vi "InitialDelayCountdown_DP_Ver1.0.vi"(1 "Temp. Display Ref Array":refnum<vi>[](array[refnum]), 9 "output cluster":T1={"Main Sweep"=0, "Steps Config:"={"total points:"=0, "Step Delay (s)"=0.0, "Ini Delay (s)"=0.0, "# of steps:"=0}, "Temperature Control (ITC 503):"={"GPIB ADR"=0, "Change Heater?"={"Heater?"=FALSE, "Heater"=0}, "Change Temp?"={"Change T?"=FALSE, "Set T (K)"=0.0}, "Cluster"={"Heat Auto?"=FALSE, "Manual Heat?"=FALSE, "Heater (%)"=0.0}, "Change PID?"={"Change PID?"=FALSE, "P"=0.0, "I"=0.0, "D"=0.0}, "Change Para?"=FALSE, "Sensor"=1}, "Temperature Control (LS 340):"={"GPIB ADR"=0, "From (K)"=0.0, "To (K)"=0.0, "Rate (K/min)"=0.0, "Delta T (0.08K)"=0.0, "Temp. Header"="", "T Display Control"={"Ch B"=FALSE, "Ch C"=FALSE, "Ch D"=FALSE}}, "Magnet Control (IPS 120-10)"={"Action"=0, "Standby (s)"=0.0, "Heater on (s)"=0.0, "Sweep Setup "=[], "GPIB ADR"=0, "Change Para?"=FALSE}, "Keithley 6221 :"=[], "Measuring Instruments : "=[], "Lock-In SR7265 :"=[], "Deascription of \nthis measurement"="", "Instruments Config:"=[], "LS372 Bridge : 2"=[{"GPIB"=0, "Excitation"=0, "Autorange?"=FALSE, "Range"=0, "Current"=0, "Voltage"=0, "DataHeader"="Rx;Ry"}], "Magnet Control (CS4) 2"={"Action"=1, "Standby (s)"=0.0, "Heater on (s)"=300.0, "Sweep Setup "=[], "GPIB ADR"=0, "Change Para?"=FALSE}} {"Magnet Control (CS4) 2"."GPIB ADR" items=["None"=0, "25"=25]; "Magnet Control (CS4) 2"."Sweep Setup"."Rate in Range (T/min)" min=0.001 max=0.5 step=0.001; "Magnet Control (CS4) 2"."Sweep Setup"."Hold(min)" min=0.0; "Magnet Control (CS4) 2"."Sweep Setup"."Set Point (T)" min=-9.0 max=9.0 step=0.001; "Magnet Control (CS4) 2"."Action" items=["Up", "Down", "Pause", "Zero"]; "LS372 Bridge : 2"."Voltage" items=["2.00 uV"=1, "6.32 uV"=2, "20.0 uV"=3, "63.2 uV"=4, "200 uV"=5, "632 uV"=6, "2.0 mV"=7, "6.32 mV"=8]; "LS372 Bridge : 2"."Current" items=["1.00 pA"=1, "3.16 pA"=2, "10.0 pA"=3, "31.6 pA"=4, "100 pA"=5, "316 pA"=6, "1.00 nA"=7, "3.16 nA"=8, "10 nA"=9, "31.6 nA"=10, "100 nA"=11, "316 nA"=12, "1.00 uA"=13, "3.16 uA"=14, "10.0 uA"=15, "31.6 uA"=16, "100 uA"=17, "316 uA"=18, "1.00 mA"=19, "3.16 mA"=20, "10.0 mA"=21, "31.6 mA"=22]; "LS372 Bridge : 2"."Range" items=["2.0 m"=1, "6.32 m"=2, "20.0 m"=3, "63.2 m"=4, "200 m"=5, "632 m"=6, "2.00"=7, "6.32"=8, "20.0"=9, "63.2"=10, "200"=11, "632"=12, "2.00 k"=13, "6.32 k"=14, "20.0 k"=15, "63.2 k"=16, "200 k"=17, "632 k"=18, "2.00 M"=19, "6.32 M"=20, "20.0 M"=21, "63.2 M"=22]; "LS372 Bridge : 2"."Excitation" items=["Voltage", "Current"]; "LS372 Bridge : 2"."GPIB" items=["None"=0, "9"=9]; "Main Sweep" items=["Time", "DC Current", "Delta Current", "Pulse Delta Current", "Sine Current", "Lock-in Vosc"]; "Temperature Control (ITC 503):"."Sensor" items=["T2", "T3"]; "Magnet Control (IPS 120-10)"."Action" items=["Hold", "To Set point", "To Zero", "Clamp"]; "Keithley 6221 :"."Sweep Mode" items=["Linear", "Log", "Exp", "Inverse", "Manual"]}, 11 "error in":errorcluster, 12 "B Field Display Tex Array":refnum<vi>[](array[refnum])) -> (4 "Stay duration pts":dbl[](array[numeric]), 8 "2D Array of DC Source or Lock-In Ctrl Run Cluster":cluster{"GPIB ADR":u16, "DC St. Pt.":dbl}[][](array[cluster]), 10 "output cluster 2":T1={"Main Sweep"=0, "Steps Config:"={"total points:"=0, "Step Delay (s)"=0.0, "Ini Delay (s)"=0.0, "# of steps:"=0}, "Temperature Control (ITC 503):"={"GPIB ADR"=0, "Change Heater?"={"Heater?"=FALSE, "Heater"=0}, "Change Temp?"={"Change T?"=FALSE, "Set T (K)"=0.0}, "Cluster"={"Heat Auto?"=FALSE, "Manual Heat?"=FALSE, "Heater (%)"=0.0}, "Change PID?"={"Change PID?"=FALSE, "P"=0.0, "I"=0.0, "D"=0.0}, "Change Para?"=FALSE, "Sensor"=1}, "Temperature Control (LS 340):"={"GPIB ADR"=0, "From (K)"=0.0, "To (K)"=0.0, "Rate (K/min)"=0.0, "Delta T (0.08K)"=0.0, "Temp. Header"="", "T Display Control"={"Ch B"=FALSE, "Ch C"=FALSE, "Ch D"=FALSE}}, "Magnet Control (IPS 120-10)"={"Action"=0, "Standby (s)"=0.0, "Heater on (s)"=0.0, "Sweep Setup "=[], "GPIB ADR"=0, "Change Para?"=FALSE}, "Keithley 6221 :"=[], "Measuring Instruments : "=[], "Lock-In SR7265 :"=[], "Deascription of \nthis measurement"="", "Instruments Config:"=[], "LS372 Bridge : 2"=[{"GPIB"=0, "Excitation"=0, "Autorange?"=FALSE, "Range"=0, "Current"=0, "Voltage"=0, "DataHeader"="Rx;Ry"}], "Magnet Control (CS4) 2"={"Action"=1, "Standby (s)"=0.0, "Heater on (s)"=300.0, "Sweep Setup "=[], "GPIB ADR"=0, "Change Para?"=FALSE}} {"Magnet Control (CS4) 2"."GPIB ADR" items=["None"=0, "25"=25]; "Magnet Control (CS4) 2"."Sweep Setup"."Rate in Range (T/min)" min=0.001 max=0.5 step=0.001; "Magnet Control (CS4) 2"."Sweep Setup"."Hold(min)" min=0.0; "Magnet Control (CS4) 2"."Sweep Setup"."Set Point (T)" min=-9.0 max=9.0 step=0.001; "Magnet Control (CS4) 2"."Action" items=["Up", "Down", "Pause", "Zero"]; "LS372 Bridge : 2"."Voltage" items=["2.00 uV"=1, "6.32 uV"=2, "20.0 uV"=3, "63.2 uV"=4, "200 uV"=5, "632 uV"=6, "2.0 mV"=7, "6.32 mV"=8]; "LS372 Bridge : 2"."Current" items=["1.00 pA"=1, "3.16 pA"=2, "10.0 pA"=3, "31.6 pA"=4, "100 pA"=5, "316 pA"=6, "1.00 nA"=7, "3.16 nA"=8, "10 nA"=9, "31.6 nA"=10, "100 nA"=11, "316 nA"=12, "1.00 uA"=13, "3.16 uA"=14, "10.0 uA"=15, "31.6 uA"=16, "100 uA"=17, "316 uA"=18, "1.00 mA"=19, "3.16 mA"=20, "10.0 mA"=21, "31.6 mA"=22]; "LS372 Bridge : 2"."Range" items=["2.0 m"=1, "6.32 m"=2, "20.0 m"=3, "63.2 m"=4, "200 m"=5, "632 m"=6, "2.00"=7, "6.32"=8, "20.0"=9, "63.2"=10, "200"=11, "632"=12, "2.00 k"=13, "6.32 k"=14, "20.0 k"=15, "63.2 k"=16, "200 k"=17, "632 k"=18, "2.00 M"=19, "6.32 M"=20, "20.0 M"=21, "63.2 M"=22]; "LS372 Bridge : 2"."Excitation" items=["Voltage", "Current"]; "LS372 Bridge : 2"."GPIB" items=["None"=0, "9"=9]; "Main Sweep" items=["Time", "DC Current", "Delta Current", "Pulse Delta Current", "Sine Current", "Lock-in Vosc"]; "Temperature Control (ITC 503):"."Sensor" items=["T2", "T3"]; "Magnet Control (IPS 120-10)"."Action" items=["Hold", "To Set point", "To Zero", "Clamp"]; "Keithley 6221 :"."Sweep Mode" items=["Linear", "Log", "Exp", "Inverse", "Manual"]}, 15 "error out":errorcluster)   [LabVIEW 2012]
doc: "Initial Delay for LS336 Temperature controller"
panel:
  in  "Initial Delay (sec)":dbl=25.0
  in  "Skip":bool
  out "Time Count down":dbl format="%02d"
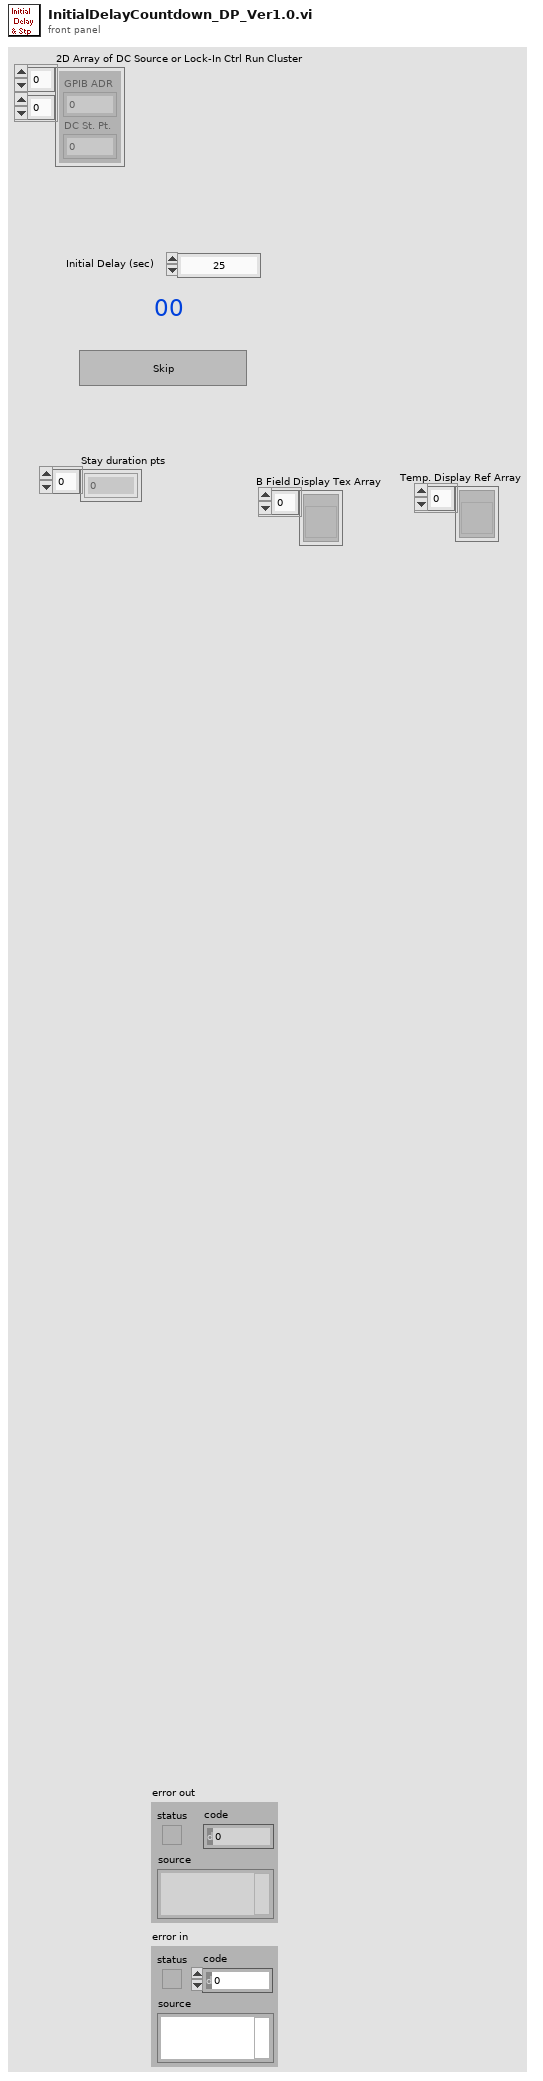
[diagram p1: front panel]
types:
  T1 = cluster{"Main Sweep":u8, "Steps Config:":cluster{"total points:":u32, "Step Delay (s)":dbl, "Ini Delay (s)":dbl, "# of steps:":u32}, "Temperature Control (ITC 503):":cluster{"GPIB ADR":u16, "Change Heater?":cluster{"Heater?":bool, "Heater":u8}, "Change Temp?":cluster{"Change T?":bool, "Set T (K)":dbl}, "Cluster":cluster{"Heat Auto?":bool, "Manual Heat?":bool, "Heater (%)":dbl}, "Change PID?":cluster{"Change PID?":bool, "P":dbl, "I":dbl, "D":dbl}, "Change Para?":bool, "Sensor":u16}, "Temperature Control (LS 340):":cluster{"GPIB ADR":u16, "From (K)":dbl, "To (K)":dbl, "Rate (K/min)":dbl, "Delta T (0.08K)":dbl, "Temp. Header":string, "T Display Control":cluster{"Ch B":bool, "Ch C":bool, "Ch D":bool}}, "Magnet Control (IPS 120-10)":cluster{"Action":u16, "Standby (s)":dbl, "Heater on (s)":dbl, "Sweep Setup ":cluster{"Set Point (T)":dbl, "Set Rate(T/min)":dbl, "Hold(min)":dbl}[], "GPIB ADR":u16, "Change Para?":bool}, "Keithley 6221 :":cluster{"Delta mode":bool, "Const I":bool, "Pulse Delta mode":bool, "Sine Wave Mode":bool, "From I_HI (A)":dbl, "From I (A)":dbl, "I_LO (A)":dbl, "From I_H (A)":dbl, "I_L (A)":dbl, "Freq (Hz)":dbl, "From I_Sin (A)":dbl, "DC Offset (A)":dbl, "Delay Time (s)":dbl, "Pulse Width (s)":dbl, "Delay (s)":dbl, "To I (A)":dbl, "ASymmetric?":bool, "To I_HI (A)":dbl, "To I_H (A)":dbl, "To I_Sin (A)":dbl, "GPIB ADR":u16, "Sweep Mode":u8, "Delta Unit":string, "2182A range (V)":dbl, "6221 Compliance (V)":dbl}[], "Measuring Instruments : ":cluster{"GPIB Bus":dbl, "GPIB Addr":dbl, "Instrument":enum16{"None", "HP34401DMM", "Lockin 7265", "HP3456/7A", "HP3478A", "HP3325FG", "Keithley2182A"}, "Instru Header":string}[], "Lock-In SR7265 :":cluster{"GPIB ADR":u16, "From":dbl, "To":dbl, "Header(;)":string, "Sweep Mode":u8}[], "Deascription of \nthis measurement":string, "Instruments Config:":string[][], "LS372 Bridge : 2":cluster{"GPIB":u16, "Excitation":u16, "Autorange?":bool, "Range":u16, "Current":u16, "Voltage":u16, "DataHeader":string}[], "Magnet Control (CS4) 2":cluster{"Action":u16, "Standby (s)":dbl, "Heater on (s)":dbl, "Sweep Setup ":cluster{"Set Point (T)":dbl, "Hold(min)":dbl, "Rate in Range (T/min)":dbl[]}[], "GPIB ADR":u16, "Change Para?":bool}}
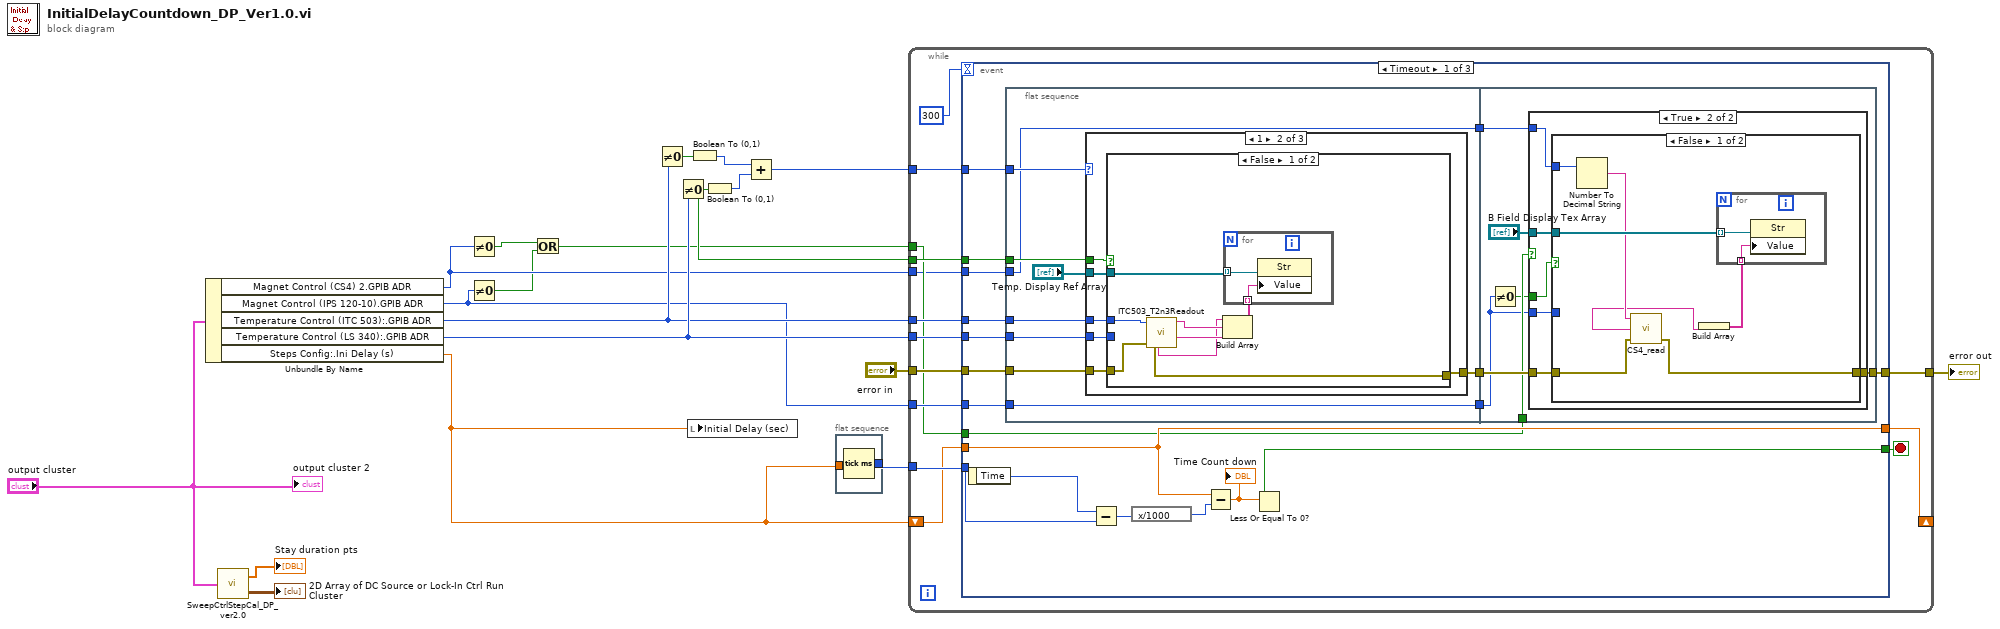
[diagram p0: block diagram]
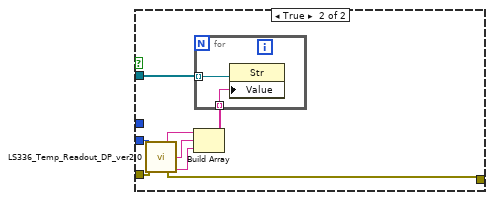
[diagram p3: hidden frame]
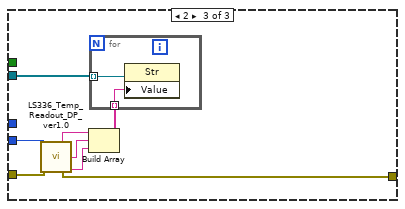
[diagram p4: hidden frame]
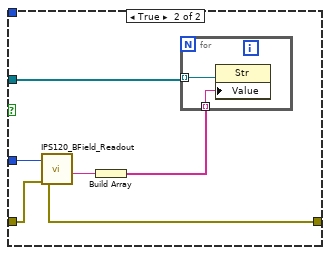
[diagram p6: hidden frame]
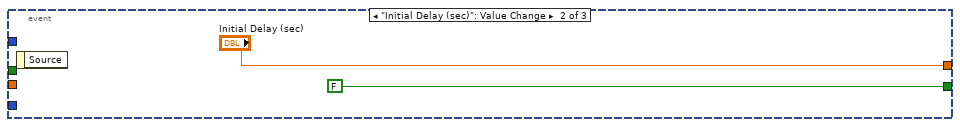
[diagram p7: hidden frame]
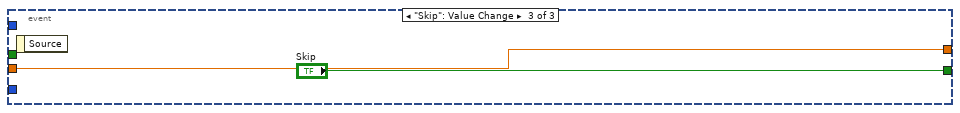
[diagram p8: hidden frame]
diagram:
  n1 = Unbundle By Name("output cluster") -> ("Magnet Control (CS4) 2.GPIB ADR"=w4:u16, "Magnet Control (IPS 120-10).GPIB ADR"=w5:u16, "Temperature Control (ITC 503):.GPIB ADR"=w8:u16, "Temperature Control (LS 340):.GPIB ADR"=w14:u16, "Steps Config:.Ini Delay (s)"=w15:dbl)
  n2 = call "SweepCtrlStepCal_DP_ver2.0.vi"("output cluster"="output cluster") -> ("Stay duration pts"=→"Stay duration pts":dbl[], "2D Array of DC Source or Lock-In Ctrl Run Cluster"=→"2D Array of DC Source or Lock-In Ctrl Run Cluster":cluster{"GPIB ADR":u16, "DC St. Pt.":dbl}[][])
  n3 = Not Equal To 0?(x=w4) -> (x != 0?=w3:bool)
  n4 = Not Equal To 0?(x=w5) -> (x != 0?=w2:bool)
  n5 = Or(x=w3, y=w2) -> (x .or. y?=w1:bool)
  n6 = Not Equal To 0?(x=w8) -> (x != 0?=w13:bool)
  n7 = Not Equal To 0?(x=w14) -> (x != 0?=w9:bool)
  n8 = local write "Initial Delay (sec)"(w15) -> ()
  n9 = Boolean To (0,1)(Boolean=w13) -> (0, 1=w11:i16)
  n10 = Boolean To (0,1)(Boolean=w9) -> (0, 1=w12:i16)
  n11 = Add(x=w11, y=w12) -> (x+y=w10:i16)
  n12 = flat-sequence {
    tunnel: [w20] -> w18
    tunnel: w15 -> [_]
    frame #0 {
      n13 = Tick Count (ms)() -> (millisecond timer value=w20:u32)
    }
  }
  n14 = while {
    tunnel: w18 -> [w34]
    shift-right: [w31] -> _
    shift-left: w15 -> [w32]
    tunnel: "error in" -> [w30]
    tunnel: [w29] -> w16
    tunnel: w14 -> [w28]
    tunnel: w10 -> [w26]
    tunnel: w9 -> [w25]
    tunnel: w8 -> [w24]
    tunnel: w5 -> [w23]
    tunnel: w4 -> [w21]
    tunnel: w1 -> [w22]
    stop <- w27 stop-if-true
    n15 = event shown="[0] Timeout" {
      selector: _ -> [_ _ _]
      dyn-events: _ -> [_ _ _]
      timeout: 300 -> [_ _ _]
      tunnel: w34 -> [w51 _ _]
      tunnel: w32 -> [w48 _ w134]
      tunnel: [w50 FALSE "Skip"] -> w27
      tunnel: [w48 "Initial Delay (sec)" w134] -> w31
      tunnel: w30 -> [w46 _ _]
      tunnel: [w40 _ _] -> w29
      tunnel: w28 -> [w45 _ _]
      tunnel: w26 -> [w44 _ _]
      tunnel: w25 -> [w43 _ _]
      tunnel: w24 -> [w42 _ _]
      tunnel: w23 -> [w39 _ _]
      tunnel: w22 -> [w37 _ _]
      tunnel: w21 -> [w36 _ _]
      event Timeout {
        n16 = event-data() -> ("Time"=w47:u32)  [unwired: 1 in]
        n17 = flat-sequence {
          tunnel: w46 -> [w62]
          tunnel: [w61] -> w41
          tunnel: w45 -> [w60]
          tunnel: w44 -> [w59]
          tunnel: w43 -> [w58]
          tunnel: w42 -> [w57]
          tunnel: w39 -> [w55]
          tunnel: [w55] -> w38
          tunnel: w36 -> [w54]
          tunnel: [w54] -> w35
          tunnel: w41 -> [w106]
          tunnel: [w105] -> w40
          tunnel: w38 -> [w102]
          tunnel: w37 -> [w103]
          tunnel: w35 -> [w100]
          frame #0 {
            n18 = case shown="1" w59 {
              tunnel: w62 -> [w63 w69 w94]
              tunnel: [w63 w68 w93] -> w61
              tunnel: w60 -> [_ w67 w92]
              tunnel: "Temp. Display Ref Array" -> [_ w66 w90]
              tunnel: w58 -> [_ w65 _]
              tunnel: w57 -> [_ w64 _]
              frame 0, Default {
              }
              frame 1 {
                n19 = case shown="False" w65 {
                  tunnel: w69 -> [w75 w84]
                  tunnel: [w74 w83] -> w68
                  tunnel: w67 -> [_ w82]
                  tunnel: w66 -> [w76 w80]
                  tunnel: w64 -> [w71 _]
                  frame False {
                    n20 = call "ITC503_T2n3Readout.vi"("GPIB Address"=w71, "error in"=w75) -> ("error out"=w74:errorcluster, "Sensor T1"=w70:string, "Sensor T2"=w73:string, "Sensor T3"=w72:string)  [unwired: 5 out]
                    n21 = Build Array(w70, w73, w72) -> (w77:string[])
                    n22 = for {
                      tunnel: w77 -> [w79] mode=indexing
                      tunnel: w76 -> [w78] mode=indexing
                      n23 = property class="Str"(reference=w78, "Value"=w79) -> ()  [unwired: 1 in, 2 out]
                    }
                  }
                  frame True {
                    n24 = call "LS336_Temp_Readout_DP_ver2.0.vi"("GPIB ADR (18)"=w82, "error in"=w84) -> ("Sensor A (K)"=w86:string, "Sensor B (K)"=w85:string, "error out"=w83:errorcluster, "Sensor C (K)"=w81:string)  [unwired: 4 in, 6 out]
                    n25 = Build Array(w86, w85, w81) -> (w87:string[])
                    n26 = for {
                      tunnel: w87 -> [w89] mode=indexing
                      tunnel: w80 -> [w88] mode=indexing
                      n27 = property class="Str"(reference=w88, "Value"=w89) -> ()  [unwired: 1 in, 2 out]
                    }
                  }
                }
              }
              frame 2 {
                n28 = call "LS336_Temp_Readout_DP_ver1.0.vi"("GPIB ADR (18)"=w92, "error in"=w94) -> ("Sensor A (K)"=w96:string, "Sensor B (K)"=w95:string, "error out"=w93:errorcluster, "Sensor C (K)"=w91:string)  [unwired: 4 in, 6 out]
                n29 = Build Array(w96, w95, w91) -> (w97:string[])
                n30 = for {
                  tunnel: w97 -> [w99] mode=indexing
                  tunnel: w90 -> [w98] mode=indexing
                  n31 = property class="Str"(reference=w98, "Value"=w99) -> ()  [unwired: 1 in, 2 out]
                }
              }
            }
          }
          frame #1 {
            n32 = Not Equal To 0?(x=w102) -> (x != 0?=w101:bool)
            n33 = case shown="True" w103 {
              tunnel: w106 -> [w107 w113]
              tunnel: [w107 w112] -> w105
              tunnel: w102 -> [_ w111]
              tunnel: "B Field Display Tex Array" -> [_ w110]
              tunnel: w101 -> [_ w109]
              tunnel: w100 -> [_ w108]
              frame False {
              }
              frame True {
                n34 = case shown="False" w109 {
                  tunnel: w113 -> [w116 w126]
                  tunnel: [w115 w125] -> w112
                  tunnel: w111 -> [_ w127]
                  tunnel: w110 -> [w120 w128]
                  tunnel: w108 -> [w118 _]
                  frame False {
                    n35 = Number To Decimal String(number=w118) -> (decimal integer string=w117:string)  [unwired: 1 in]
                    n36 = call "CS4_read.vi"("error in"=w116, "address string"=w117) -> ("error out"=w115:errorcluster, "Real Field"=w114:string)  [unwired: 2 out]
                    n37 = Build Array(w114) -> (w119:string[])
                    n38 = for {
                      tunnel: w119 -> [w122] mode=indexing
                      tunnel: w120 -> [w121] mode=indexing
                      n39 = property class="Str"(reference=w121, "Value"=w122) -> ()  [unwired: 1 in, 2 out]
                    }
                  }
                  frame True {
                    n40 = call "IPS120_BField_Readout.vi"("error in"=w126, "GPIB Address"=w127) -> ("B field read"=w124:string, "error out"=w125:errorcluster)  [unwired: 1 in, 3 out]
                    n41 = Build Array(w124) -> (w123:string[])
                    n42 = for {
                      tunnel: w123 -> [w130] mode=indexing
                      tunnel: w128 -> [w129] mode=indexing
                      n43 = property class="Str"(reference=w129, "Value"=w130) -> ()  [unwired: 1 in, 2 out]
                    }
                  }
                }
              }
            }
          }
        }
        n44 = Subtract(x=w47, y=w51) -> (x-y=w53:u32)
        n45 = expression code="x/1000"(w53) -> (w52:u32)
        n46 = Subtract(x=w48, y=w52) -> (x-y=w49:dbl)
        "Time Count down" <- w49
        n47 = Less Or Equal To 0?(x=w49) -> (x <= 0?=w50:bool)
      }
      event "Initial Delay (sec)": Value Change {
        n48 = event-data() -> ()  [unwired: 1 in, 1 out]
      }
      event "Skip": Value Change {
        n49 = event-data() -> ()  [unwired: 1 in, 1 out]
      }
    }
  }
  "error out" <- w16
  "output cluster 2" <- "output cluster"
